vi "48-bit Adder using DSP48E.vi"(8 "Input Valid":bool=TRUE, 10 "B":fxp<+/-,48,48>, 11 "A":fxp<+/-,48,48>) -> (0 "Output Valid":bool=TRUE, 3 "A+B":fxp<+/-,49,49>)   [LabVIEW 2011]
doc: "This VI adds two 48-bit numbers using DSP48E. The output is a 49-bit and carryout logic of DSP48E is used for this purpose."
uses:
  <vilib>/rvi/FXPMathLib/basic elements/DSP48E/simVIs/niFpgaDsp48eRegisters.ctl
  <vilib>/rvi/FXPMathLib/basic elements/DSP48E/simVIs/niFpgaDsp48eEnables.ctl
  <vilib>/rvi/FXPMathLib/basic elements/DSP48E/simVIs/niFpgaDsp48eResets.ctl
  <vilib>/rvi/FXPMathLib/basic elements/DSP48E/simVIs/niFpgaDsp48eSimulationState.ctl
  <vilib>/rvi/FXPMathLib/basic elements/DSP48E/subVIs/niFpgaDsp48eType.ctl
  <vilib>/rvi/FXPMathLib/basic elements/DSP48E/subVIs/niFpgaDsp48eAlumodeOpmodeCarryinselState.ctl
  <vilib>/rvi/FXPMathLib/basic elements/DSP48E/subVIs/niFpgaDsp48eUseMultiplierState.ctl
  <vilib>/rvi/FXPMathLib/basic elements/DSP48E/subVIs/niFpgaDsp48eLogicUnitModeState.ctl
  <vilib>/rvi/FXPMathLib/basic elements/DSP48E/subVIs/niFpgaDsp48eSelectPatternState.ctl
  <vilib>/rvi/FXPMathLib/basic elements/DSP48E/subVIs/niFpgaDsp48eSelectMaskState.ctl
  <vilib>/rvi/FXPMathLib/basic elements/DSP48E/subVIs/niFpgaDsp48eAutoresetState.ctl
  <vilib>/rvi/FXPMathLib/basic elements/DSP48E/simVIs/niFpgaDsp48eSimMultiplier.vi
  <vilib>/rvi/FXPMathLib/basic elements/DSP48E/simVIs/niFpgaDsp48eSimArithmetic.vi
  <vilib>/rvi/FXPMathLib/basic elements/DSP48E/simVIs/niFpgaDsp48eSimPatternDetect.vi
  <vilib>/rvi/FXPMathLib/basic elements/DSP48E/simVIs/niFpgaDsp48eSimP.vi
  <vilib>/rvi/FXPMathLib/basic elements/DSP48E/simVIs/niFpgaDsp48eSimUpdateState.vi
  <vilib>/rvi/FXPMathLib/basic elements/DSP48E/simVIs/niFpgaDsp48eCheckMode.vi
  <vilib>/rvi/FXPMathLib/basic elements/DSP48E/simVIs/niFpgaDsp48eReportInvalidMode.vi
  <vilib>/rvi/FXPMathLib/basic elements/FxpDiscreteDelay/XNode/nifxpmath_DiscreteDelay.xnode
  <vilib>/rvi/FXPMathLib/basic elements/DSP48E/XNode/niFpgaDsp48e.xnode
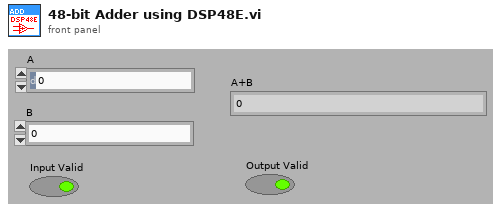
[diagram p1: front panel]
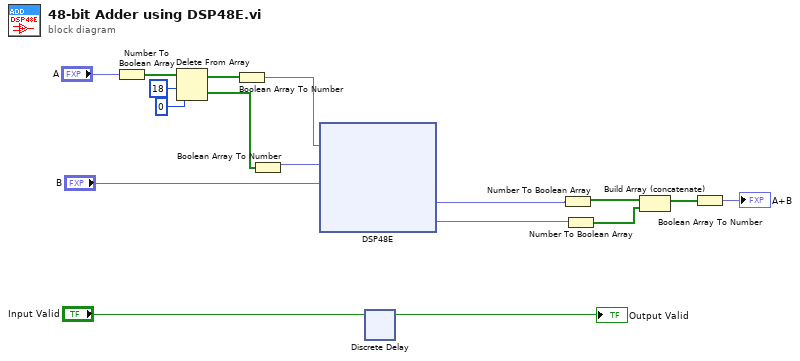
[diagram p0: block diagram]
diagram:
  n1 = Number To Boolean Array(number="A") -> (Boolean array=w5:bool[])
  n2 = Delete From Array(array=w5, length=18, index=0) -> (deleted portion=w3:bool[], array with subset deleted=w4:bool[])
  n3 = Boolean Array To Number(Boolean array=w4) -> (number=w12:fxp<+/-,30,30>)
  n4 = Boolean Array To Number(Boolean array=w3) -> (number=w13:fxp<+/-,18,18>)
  n5 = xnode "DSP48E"("a"=w12, "b"=w13, "c"="B") -> ("p"=w11:fxp<+/-,48,48>, "carryout"=w10:fxp<+,4,4>)
  n6 = xnode "Discrete Delay"("D"="Input Valid") -> ("Q"=→"Output Valid":bool)
  n7 = Number To Boolean Array(number=w11) -> (Boolean array=w9:bool[])
  n8 = Number To Boolean Array(number=w10) -> (Boolean array=w8:bool[])
  n9 = Build Array (concatenate)(w9, w8) -> (w7:bool[])
  n10 = Boolean Array To Number(Boolean array=w7) -> (number=→"A+B":fxp<+/-,49,49>)
